vi "Get Tweets Search Old.vi"(8 "error in":errorcluster, 9 "Tweets to Read (10)":i32=10 min=0 max=200 step=1, 10 "Query":string="#LVHacker", 11 "Twitter Handle In":T1={"OAuth Credentials"={"Signature Method"=enum."HMAC-SHA1", "Version"="1.0", "Client"={"Token"="", "Secret"=""}, "Access"={"Token"="", "Secret"=""}}, "since ID"="", "max ID"="", "Screen Name"=""}) -> (0 "error out":errorcluster, 1 "Actual Num of Tweets Read":i32, 2 "Old Tweets Read":T5[](array[typedef]), 3 "Twitter Handle Out":T1={"OAuth Credentials"={"Signature Method"=enum."HMAC-SHA1", "Version"="1.0", "Client"={"Token"="", "Secret"=""}, "Access"={"Token"="", "Secret"=""}}, "since ID"="", "max ID"="", "Screen Name"=""}, 5 "Time Stamp of Oldest Tweet":timestamp)   [LabVIEW 2011, in "i3-twitter.lvlib"]
doc: "Use this VI to search for Tweets based on a <b>Search Query</b>. A common Search Query may be a hashtag search such as #LVHacker. <b>Get Tweets Search New.vi</b> returns new Tweets for the authenticated user since the last time this function was called with the <b>Twitter Handle</b>.\n\nThe first time the function is called it returns the number of Tweets specified by <b>Tweets to Read</b> and each consecutive call returns Tweets that have been received after the <b>Time Stamp of Newest Tweet</b>."
uses:
  i3-twitter.lvlib
  Controls/Tweet.ctl
  Controls/Twitter Handle.ctl
  i3-oauth/Controls/OAuth Handle.ctl
  i3-oauth/Controls/Signature Method.ctl
  i3-oauth/Controls/Credentials.ctl
  i3-oauth/Controls/HTTP Method.ctl
  i3-json/JSON Parsing/Get Object Parameter Files/Get Object Parameter - Object.vi
  i3-json/JSON Parsing/Get Array Value at Index Files/Get Array Value at Index - Object.vi
  i3-json/JSON Parsing/Get Object Parameter Files/Get Object Parameter - String.vi
  i3-oauth/i3-oauth.lvlib
  <vilib>/httpClient/LabVIEWHTTPClient.lvlib
  i3-json/i3-json.lvlib
panel:
  out "Full URL":string
  out "body":string
  out "headers":string
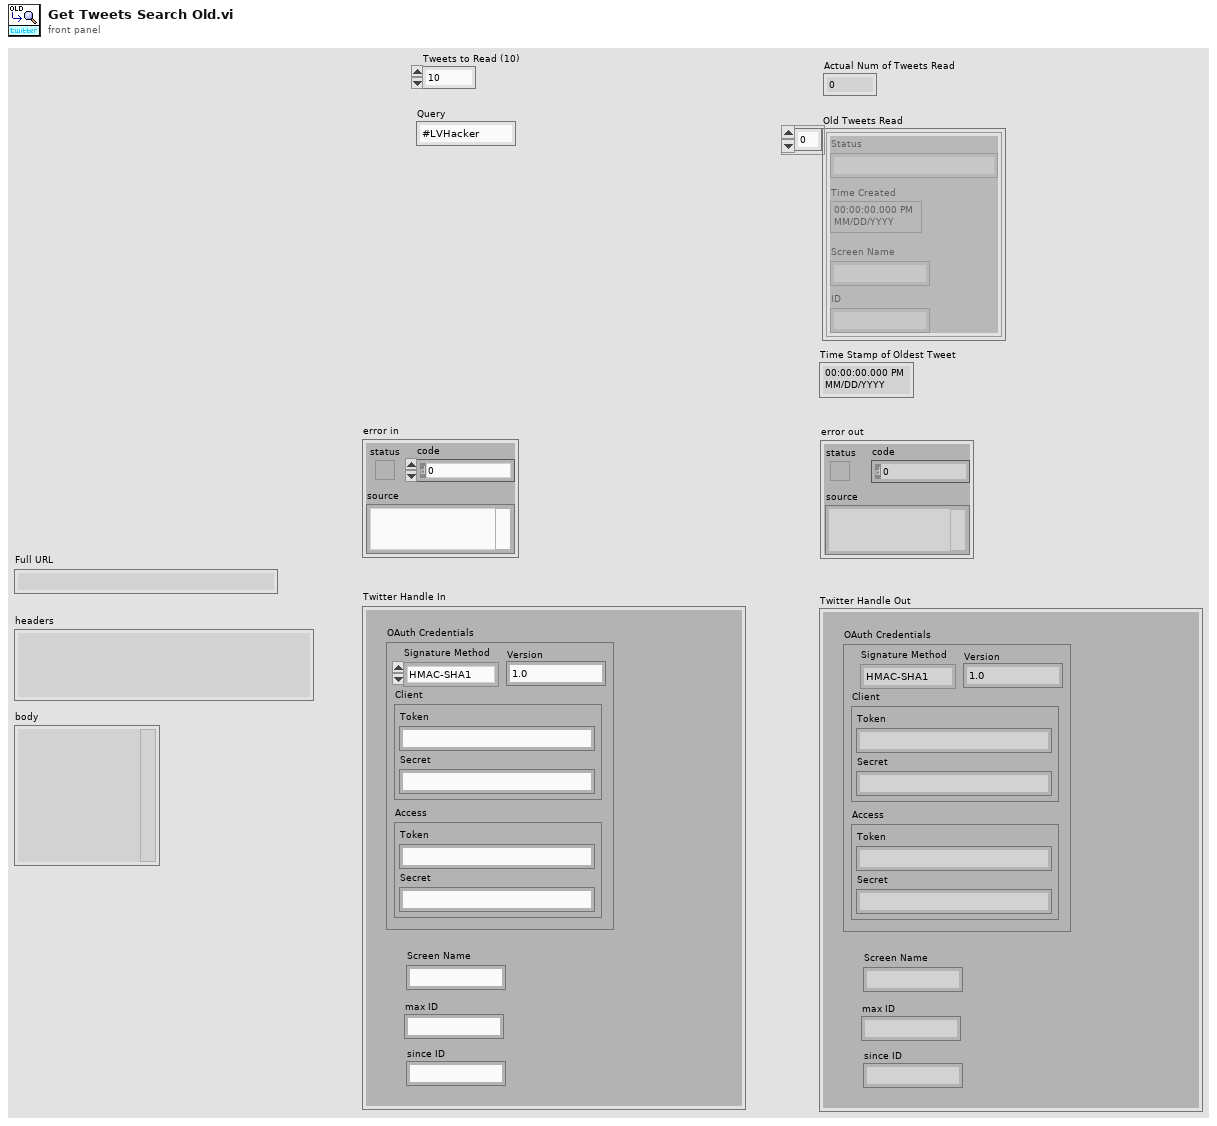
[diagram p1: front panel]
types:
  T1 = typedef "i3-twitter.lvlib/Twitter Handle.ctl" = cluster{"OAuth Credentials":T2, "since ID":string, "max ID":string, "Screen Name":string}
  T2 = typedef "i3-oauth.lvlib/OAuth Handle.ctl" = cluster{"Signature Method":T3, "Version":string, "Client":T4, "Access":T4}
  T3 = typedef "i3-oauth.lvlib/Signature Method.ctl" = enum16{"HMAC-MD5", "HMAC-SHA1", "HMAC-SHA224", "HMAC-SHA256", "HMAC-SHA384", "HMAC-SHA512"}
  T4 = typedef "i3-oauth.lvlib/Credentials.ctl" = cluster{"Token":string, "Secret":string}
  T5 = typedef "i3-twitter.lvlib/Tweet.ctl" = cluster{"Status":string, "Time Created":timestamp, "Screen Name":string, "ID":string}
  T6 = typedef "i3-oauth.lvlib/HTTP Method.ctl" = enum16{"GET", "POST", "PUT", "DELETE"}
  T7 = typedef "i3-oauth.lvlib/Name-Value Pair.ctl" = cluster{"Name":string, "Value":string}
  T8 = typedef "LabVIEWHTTPClient.lvlib/ClientHandle.ctl" = refnum<k1>
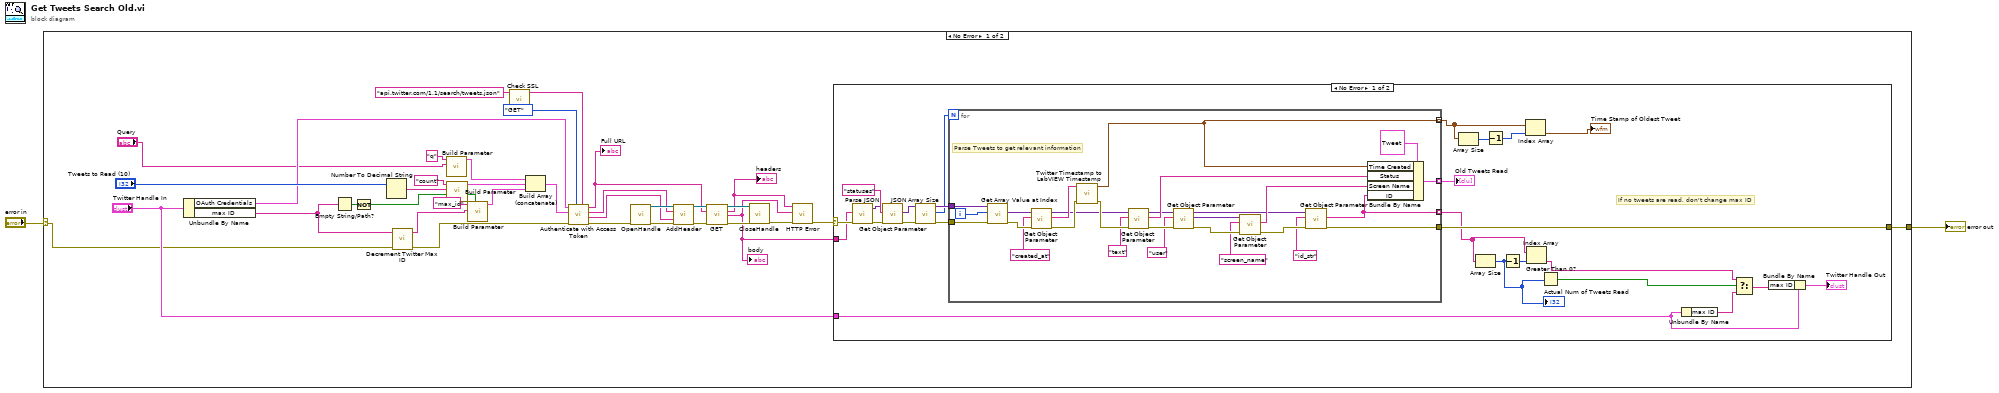
[diagram p0: block diagram]
diagram:
  n1 = case shown="No Error" "error in" {
    selector: "error in" -> [w5 w92]
    tunnel: [w21 w92] -> w2
    frame No Error {
      n2 = Unbundle By Name("Twitter Handle In") -> ("OAuth Credentials"=w18:T2, "max ID"=w4:string)
      n3 = Empty String/Path?(string/path=w4) -> (empty?=w9:bool)
      n4 = Not(x=w9) -> (.not. x?=w8:bool)
      n5 = Number To Decimal String(number="Tweets to Read (10)") -> (decimal integer string=w27:string)  [unwired: 1 in]
      n6 = call "Decrement Twitter Max ID.vi"("error in (no error)"=w5, "ID In"=w4) -> ("error out"=w6:errorcluster, "ID Out"=w3:string)  [unwired: 8 in]
      n7 = call "Build Parameter.vi"("Value"="Query", "Key"="q") -> ("Parameter Array"=w12:T7[])  [unwired: 9 in]
      n8 = call "Build Parameter.vi"("Value"=w27, "Key"="count") -> ("Parameter Array"=w15:T7[])  [unwired: 9 in]
      n9 = call "Build Parameter.vi"("Return Parameter? (T)"=w8, "Value"=w3, "Key"="max_id") -> ("Parameter Array"=w7:T7[])  [unwired: 8 in]
      n10 = call "Check SSL.vi"("Input URL"="api.twitter.com/1.1/search/tweets.json" ("Base URL")) -> ("Output URL"=w16:string)  [unwired: 8 in]
      n11 = Build Array (concatenate)(w12, w15, w7) -> (w26:T7[])
      n12 = call "Authenticate with Access Token.vi"("Base URL"=w16, "HTTP Method"=HTTP_Method."GET", "error in (no error)"=w6, "URL Parameters"=w26, "OAuth Handle"=w18) -> ("error out"=w25:errorcluster, "Header Value"=w31:string, "Header Parameter"=w32:string, "Full URL"=w30:string)  [unwired: 2 in, 1 out]
      "Full URL" <- w30
      n13 = call <vilib>:"OpenHandle.vi"("error in (no error)"=w25) -> ("client handle out"=w38:T8, "error out"=w37:errorcluster)  [unwired: 13 in]
      n14 = call <vilib>:"AddHeader.vi"("client handle"=w38, "header"=w32, "value"=w31, "error in (no error)"=w37) -> ("client handle out"=w36:T8, "error out"=w35:errorcluster)  [unwired: 10 in]
      n15 = call <vilib>:"GET.vi"("client handle"=w36, "url"=w30, "error in (no error)"=w35) -> ("client handle out"=w34:T8, "headers"=w24:string, "body"=w20:string, "error out"=w33:errorcluster)  [unwired: 9 in]
      "body" <- w20
      "headers" <- w24
      n16 = call <vilib>:"CloseHandle.vi"("client handle"=w34, "error in (no error)"=w33) -> ("error out"=w23:errorcluster)  [unwired: 13 in]
      n17 = call "HTTP Error.vi"("error in (no error)"=w23, "Body"=w20, "Header"=w24) -> ("error out"=w22:errorcluster)  [unwired: 6 in, 2 out]
      n18 = case shown="No Error" w22 {
        selector: w22 -> [w59 w91]
        tunnel: [w58 w91] -> w21
        tunnel: w20 -> [w57 _]
        tunnel: "Twitter Handle In" -> [w47 _]
        frame No Error {
          # "If no tweets are read, don't change max ID"
          n19 = call "Parse JSON.vi"("error in (no error)"=w59, "JSON String"=w57) -> ("error out"=w52:errorcluster, "JSON Tree"=w53:variant)  [unwired: 6 in, 2 out]
          n20 = call-poly "Get Object Parameter.vi"("error in (no error)"=w52, "Parameter Name"="statuses", "JSON Tree In (JSON Object)"=w53) -> ("error out"=w56:errorcluster, "JSON Object"=w55:variant)  [unwired: 5 in, 2 out]
          n21 = call "JSON Array Size.vi"("error in (no error)"=w56, "JSON Tree In (JSON Array)"=w55) -> ("error out"=w61:errorcluster, "Array Size"=w62:i32, "JSON Tree Passthrough (JSON Array)"=w63:variant)  [unwired: 7 in]
          n22 = for {
            N: w62 -> [_]
            tunnel: w61 -> [w74]
            tunnel: [w77] -> w60 mode=indexing
            tunnel: [w76] -> w58
            tunnel: w63 -> [w73]
            tunnel: [w72] -> w43 mode=indexing
            tunnel: [w64] -> w41 mode=indexing
            i -> [w79]
            # "Parse Tweets to get relevant information"
            n23 = call-poly "Get Array Value at Index.vi"("error in (no error)"=w74, "Index"=w79, "JSON Tree In (JSON Array)"=w73) -> ("error out"=w86:errorcluster, "JSON Object"=w70:variant)  [unwired: 5 in, 2 out]
            n24 = call-poly "Get Object Parameter.vi"("error in (no error)"=w86, "Parameter Name"="created_at", "JSON Tree In (JSON Object)"=w70) -> ("error out"=w69:errorcluster, "String Value"=w68:string, "JSON Tree Out Passthrough"=w67:variant)  [unwired: 5 in, 1 out]
            n25 = call "Twitter Timestamp to LabVIEW Timestamp.vi"("error in"=w69, "Twitter Time Stamp"=w68) -> ("error out"=w87:errorcluster, "LabVIEW Time Stamp"=w72:timestamp)  [unwired: 6 in]
            n26 = call-poly "Get Object Parameter.vi"("error in (no error)"=w87, "Parameter Name"="text", "JSON Tree In (JSON Object)"=w67) -> ("error out"=w88:errorcluster, "String Value"=w75:string, "JSON Tree Out Passthrough"=w66:variant)  [unwired: 5 in, 1 out]
            n27 = call-poly "Get Object Parameter.vi"("error in (no error)"=w88, "Parameter Name"="user", "JSON Tree In (JSON Object)"=w66) -> ("error out"=w89:errorcluster, "JSON Object"=w71:variant, "JSON Tree Out Passthrough"=w65:variant)  [unwired: 5 in, 1 out]
            n28 = call-poly "Get Object Parameter.vi"("error in (no error)"=w89, "Parameter Name"="screen_name", "JSON Tree In (JSON Object)"=w71) -> ("error out"=w90:errorcluster, "String Value"=w82:string)  [unwired: 5 in, 2 out]
            n29 = call-poly "Get Object Parameter.vi"("error in (no error)"=w90, "Parameter Name"="id_str", "JSON Tree In (JSON Object)"=w65) -> ("error out"=w76:errorcluster, "String Value"=w64:string)  [unwired: 5 in, 2 out]
            n30 = Bundle By Name(cluster=T5 {"Status"="", "Time Created"=timestamp(0 s since 1904-01-01), "Screen Name"="", "ID"=""}, "Time Created"=w72, "Status"=w75, "Screen Name"=w82, "ID"=w64) -> (w77:T5)
          }
          "Old Tweets Read" <- w60
          n31 = Array Size(array=w43) -> (size(s)=w46:i32)
          n32 = Array Size(array=w41) -> (size(s)=w39:i32)
          "Actual Num of Tweets Read" <- w39
          n33 = Decrement(x=w46) -> (x-1=w45:i32)
          n34 = Decrement(x=w39) -> (x-1=w42:i32)
          n35 = Index Array(array=w43, index=w45) -> (element=→"Time Stamp of Oldest Tweet":timestamp)
          n36 = Index Array(array=w41, index=w42) -> (element=w40:string)
          n37 = Greater Than 0?(x=w39) -> (x > 0?=w51:bool)
          n38 = Unbundle By Name(w47) -> ("max ID"=w48:string)
          n39 = Select(t=w40, s=w51, f=w48) -> (s? t:f=w50:string)
          n40 = Bundle By Name(cluster=w47, "max ID"=w50) -> (→"Twitter Handle Out":T1)
        }
        frame Error {
        }
      }
    }
    frame Error {
    }
  }
  "error out" <- w2
